vi "Close.vi"(0 "SLSC Interface in":refnum<class "SLSC Interface.lvclass">, 11 "error in (no error)":errorcluster) -> (15 "error out":errorcluster)   [LabVIEW 2015, in "SLSC Interface.lvclass"]
uses:
  SLSC Interface.lvclass
  <vilib>/SLSC/Close Session.vi
  <vilib>/SLSC/SLSC.lvlib
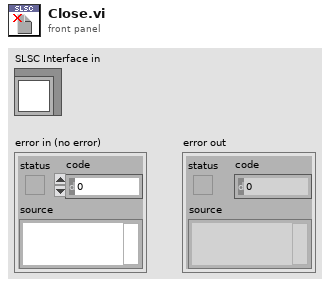
[diagram p1: front panel]
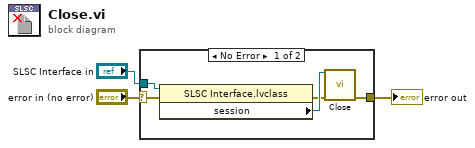
[diagram p0: block diagram]
diagram:
  n1 = case shown="No Error" "error in (no error)" {
    selector: "error in (no error)" -> [w5 w9]
    tunnel: [w8 w9] -> w2
    tunnel: "SLSC Interface in" -> [w7 _]
    frame No Error {
      n2 = property class="SLSC Interface.lvclass"(reference=w7, error in=w5) -> (error out=w4:errorcluster, "session"=w6:refnum<k21>)  [unwired: 1 out]
      n3 = call-poly <vilib>:"Close.vi"("session in"=w6, "error in (no error)"=w4) -> ("error out"=w8:errorcluster)  [unwired: 13 in]
    }
    frame Error {
    }
  }
  "error out" <- w2
